vi "Split_String.vi"(10 "Delim Char":string, 11 "Text In":string) -> (2 "Invalid Delim":bool, 3 "Splits Out":string[](array[string]))   [LabVIEW 2017]
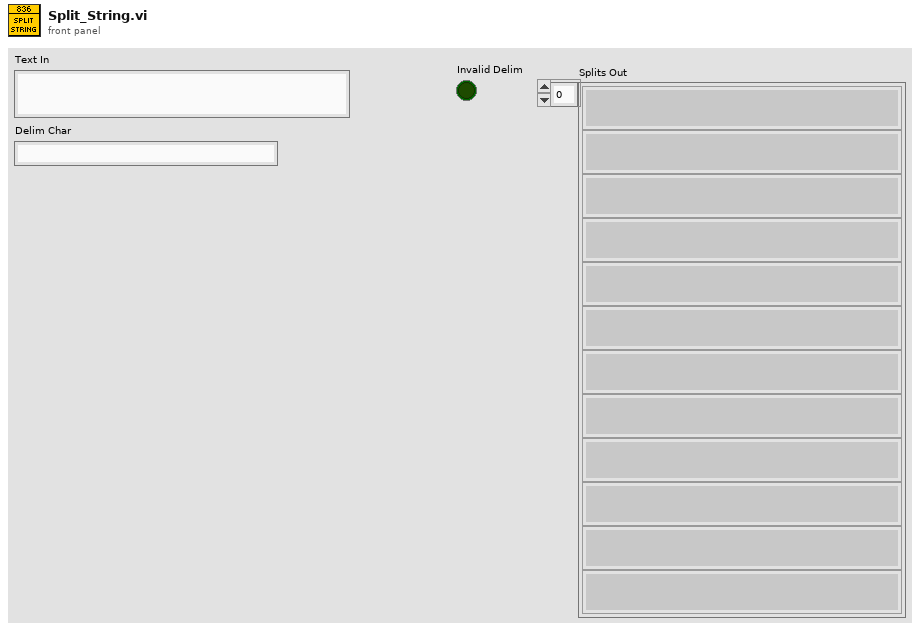
[diagram p1: front panel]
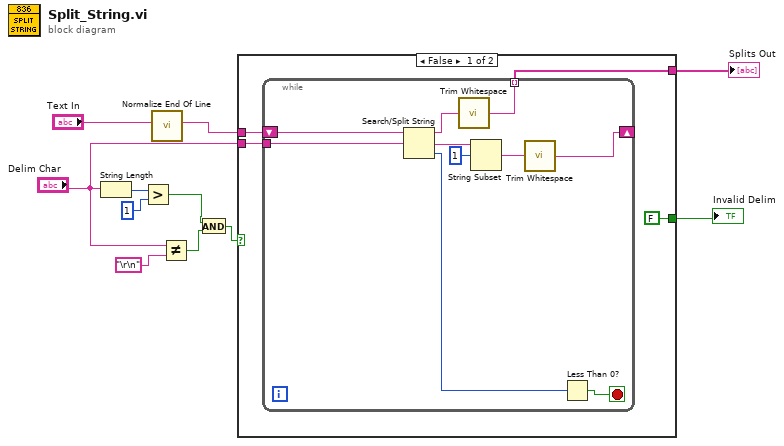
[diagram p0: block diagram]
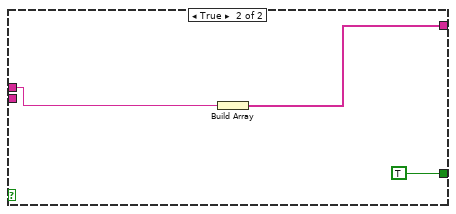
[diagram p2: hidden frame]
diagram:
  n1 = String Length(string="Delim Char") -> (length=w10:i32)
  n2 = Greater?(x=w10, y=1) -> (0:w6:bool)
  n3 = call <vilib>:"Normalize End Of Line.vi"("string in"="Text In") -> ("string out"=w1:string)  [unwired: 7 in]
  n4 = Not Equal?(x="Delim Char", y="\r\n") -> (x != y?=w3:bool)
  n5 = And(x=w6, y=w3) -> (x .and. y?=w5:bool)
  n6 = case shown="False" w5 {
    tunnel: w1 -> [w15 w28]
    tunnel: [w12 w27] -> w8
    tunnel: [FALSE TRUE] -> w7
    tunnel: "Delim Char" -> [w13 _]
    frame False {
      n7 = while {
        shift-right: [w18] -> _
        shift-left: w15 -> [w25]
        tunnel: w13 -> [w22]
        tunnel: [w16] -> w12 mode=indexing
        stop <- w24 stop-if-true
        n8 = Search/Split String(string=w25, search string/char (-)=w22) -> (substring before match=w17:string, match + rest of string=w21:string, offset of match=w23:i32)  [unwired: 1 in]
        n9 = call <vilib>:"Trim Whitespace.vi"("string"=w17) -> ("trimmed string"=w16:string)  [unwired: 1 in]
        n10 = String Subset(string=w21, offset (0)=1) -> (substring=w19:string)  [unwired: 1 in]
        n11 = call <vilib>:"Trim Whitespace.vi"("string"=w19) -> ("trimmed string"=w18:string)  [unwired: 1 in]
        n12 = Less Than 0?(x=w23) -> (x < 0?=w24:bool)
      }
    }
    frame True {
      n13 = Build Array(w28) -> (w27:string[])
    }
  }
  "Splits Out" <- w8
  "Invalid Delim" <- w7
